vi "Create or Replace File.vi"(8 "error in":errorcluster, 10 "Log File Base Path":path) -> (0 "error out":errorcluster, 2 "File Path":path, 3 "Refnum out":refnum<k34>)   [LabVIEW 2025, in "Logger.lvlib"]
doc: "Create or replace the log file at the specified location.\n_____\nBased on DQMH Dev Tools: Project Template 7.1.0.1503."
uses:
  Logger.lvlib
  <vilib>/Utility/error.llb/Trim Whitespace One-Sided.vi
  Settings Editor/Settings Editor.lvlib
  Settings Editor/Test Meta Data.ctl
panel:
  out "Settings.Meta Data":T1
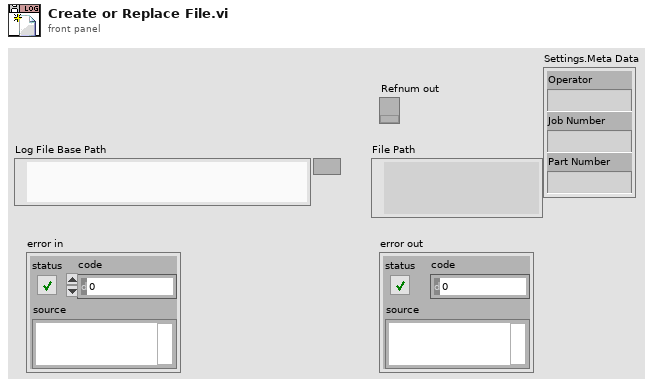
[diagram p1: front panel]
types:
  T1 = typedef "Test Meta Data.ctl" = cluster{"Operator":string, "Job Number":string, "Part Number":string}
  T2 = enum16{"open", "open or create", "create or replace", "create", "open (read-only)"}
  T3 = typedef "Settings Editor.lvlib/Update Application Settings (Reply Payload)--cluster.ctl" = cluster{"Settings":T4, "error":errorcluster}
  T4 = typedef "Settings Editor.lvlib/Settings--cluster.ctl" = cluster{"Log File Base Path":path, "Meta Data":T1}
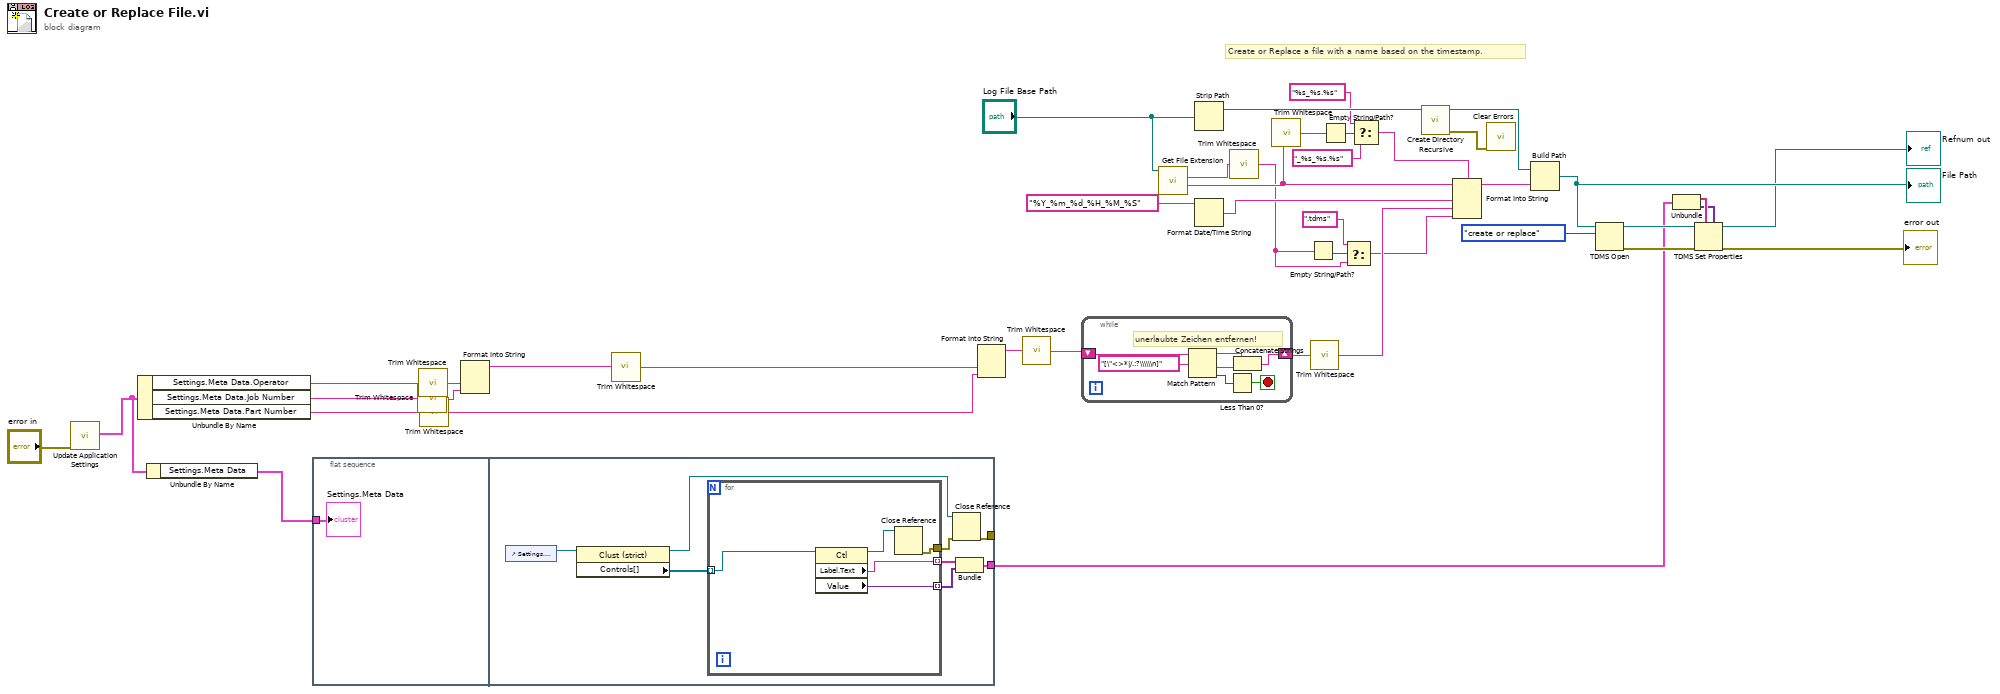
[diagram p0: block diagram]
diagram:
  # "Create or Replace a file with a name based on the timestamp."
  n1 = call "Update Application Settings.vi"("error in"="error in") -> ("Reply Payload"=w16:T3)  [unwired: 8 in, 2 out]
  n2 = Unbundle By Name(w16) -> ("Settings.Meta Data.Operator"=w19:string, "Settings.Meta Data.Job Number"=w18:string, "Settings.Meta Data.Part Number"=w17:string)
  n3 = Unbundle By Name(w16) -> ("Settings.Meta Data"=w15:T1)
  n4 = flat-sequence {
    tunnel: w15 -> [w43]
    tunnel: [w46] -> _
    tunnel: [w44] -> w14
    frame #0 {
      "Settings.Meta Data" <- w43
    }
    frame #1 {
      n5 = control-ref of="Settings.Meta Data"() -> (w51:refnum<vi>)
      n6 = property class="Clust (strict)"(reference=w51) -> (reference out=w45:refnum<vi>, "Controls[]"=w50:refnum<vi>[])  [unwired: 1 in, 1 out]
      n7 = for {
        tunnel: w50 -> [w56] mode=indexing
        tunnel: [w55] -> w49 mode=indexing
        tunnel: [w54] -> w48 mode=indexing
        tunnel: [w52] -> w47
        n8 = property class="Ctl"(reference=w56) -> (reference out=w53:refnum<vi>, "Label.Text"=w54:string, "Value"=w55:variant)  [unwired: 1 in, 1 out]
        n9 = Close Reference(reference=w53) -> (error out=w52:errorcluster)  [unwired: 1 in]
      }
      n10 = Close Reference(reference=w45, error in (no error)=w47) -> (error out=w46:errorcluster)
      n11 = Bundle(w48, w49) -> (w44:cluster{string[], variant[]})  [unwired: 1 in]
    }
  }
  n12 = call <vilib>:"Trim Whitespace.vi"("string"=w18) -> ("trimmed string"=w32:string)  [unwired: 1 in]
  n13 = call <vilib>:"Trim Whitespace.vi"("string"=w19) -> ("trimmed string"=w33:string)  [unwired: 1 in]
  n14 = call <vilib>:"Trim Whitespace.vi"("string"=w17) -> ("trimmed string"=w29:string)  [unwired: 1 in]
  n15 = Format Into String(w33, w32) -> (resulting string=w31:string)  [unwired: 3 in, 1 out]
  n16 = call <vilib>:"Trim Whitespace.vi"("string"=w31) -> ("trimmed string"=w30:string)  [unwired: 1 in]
  n17 = Format Into String(w30, w29) -> (resulting string=w28:string)  [unwired: 3 in, 1 out]
  n18 = call <vilib>:"Trim Whitespace.vi"("string"=w28) -> ("trimmed string"=w27:string)  [unwired: 1 in]
  n19 = while {
    shift-right: [w58] -> w26
    shift-left: w27 -> [w57]
    stop <- w59 stop-if-true
    # "unerlaubte Zeichen entfernen!"
    n20 = Match Pattern(string=w57, regular expression="[\"<>*|/.:?\\\\\\n]") -> (before substring=w62:string, after substring=w61:string, offset past match=w60:i32)  [unwired: 2 out]
    n21 = Less Than 0?(x=w60) -> (x < 0?=w59:bool)
    n22 = Concatenate Strings(w62, w61) -> (w58:string)
  }
  n23 = call <vilib>:"Get File Extension.vi"("file"="Log File Base Path") -> ("filename without extension"=w11:string, "lowercase file extension"=w3:string)  [unwired: 6 in, 3 out]
  n24 = Strip Path(path="Log File Base Path") -> (stripped path=w36:path)  [unwired: 1 out]
  n25 = Format Date/Time String(time format string (%c)="%Y_%m_%d_%H_%M_%S") -> (date/time string=w40:string)  [unwired: 2 in]
  n26 = call <vilib>:"Trim Whitespace.vi"("string"=w3) -> ("trimmed string"=w1:string)  [unwired: 1 in]
  n27 = call <vilib>:"Trim Whitespace.vi"("string"=w11) -> ("trimmed string"=w5:string)  [unwired: 1 in]
  n28 = Empty String/Path?(string/path=w1) -> (empty?=w6:bool)
  n29 = call <vilib>:"Trim Whitespace.vi"("string"=w26) -> ("trimmed string"=w25:string)  [unwired: 1 in]
  n30 = Empty String/Path?(string/path=w5) -> (empty?=w10:bool)
  n31 = Select(t=".tdms", s=w6, f=w1) -> (s? t:f=w2:string)
  n32 = Select(t="%s_%s.%s", s=w10, f="_%s_%s.%s") -> (s? t:f=w9:string)
  n33 = call <vilib>:"Create Directory Recursive.vi"("directory"=w36) -> ("error out"=w24:errorcluster, "directory copy"=w35:path)  [unwired: 4 in, 1 out]
  n34 = Format Into String(format string=w9, initial string=w11, w40, w25, w2) -> (resulting string=w41:string)  [unwired: 1 in, 1 out]
  n35 = call <vilib>:"Clear Errors.vi"("error in (no error)"=w24) -> ()  [unwired: 5 in, 2 out]
  n36 = Build Path(base path=w35, name or relative path=w41) -> (appended path=w37:path)
  "File Path" <- w37
  n37 = TDMS Open(10:T2."create or replace" ("operation (0:open)"), 11:w37) -> (0:w23:errorcluster, 3:w21:refnum<k34>)  [unwired: 5 in]
  n38 = Unbundle(w14) -> (w13:string[], w12:variant[])
  n39 = TDMS Set Properties(5:w12, 7:w13, 8:w23, 11:w21) -> (0:→"error out":errorcluster, 3:→"Refnum out":refnum<k34>)  [unwired: 2 in, 2 out]
